vi "Undistort (Greyscale).vi"(6 "Camera Parameters":T1, 8 "error in (no error)":errorcluster, 10 "Greyscale Image Destination":T4, 11 "Greyscale Image Source":T4) -> (0 "error out":errorcluster, 3 "Greyscale Image Destination (duplicate)":T4)   [LabVIEW 2020, in "g_ar_toolkit.image.lvlib"]
uses:
  g_ar_toolkit.image.lvlib
  Greyscale Image.ctl
  g_ar_toolkit.common/Camera Parameters.ctl
  g_ar_toolkit.common/Camera Matrix.ctl
  g_ar_toolkit.common/Camera Distortion Coefficients.ctl
  88690800-d834-48c3-9c45-44dd73aae051.vi
  g_ar_toolkit.common/Module Path.vi
  <vilib>/Utility/error.llb/Error Cluster From Error Code.vi
  g_ar_toolkit.common/g_ar_toolkit.common.lvlib
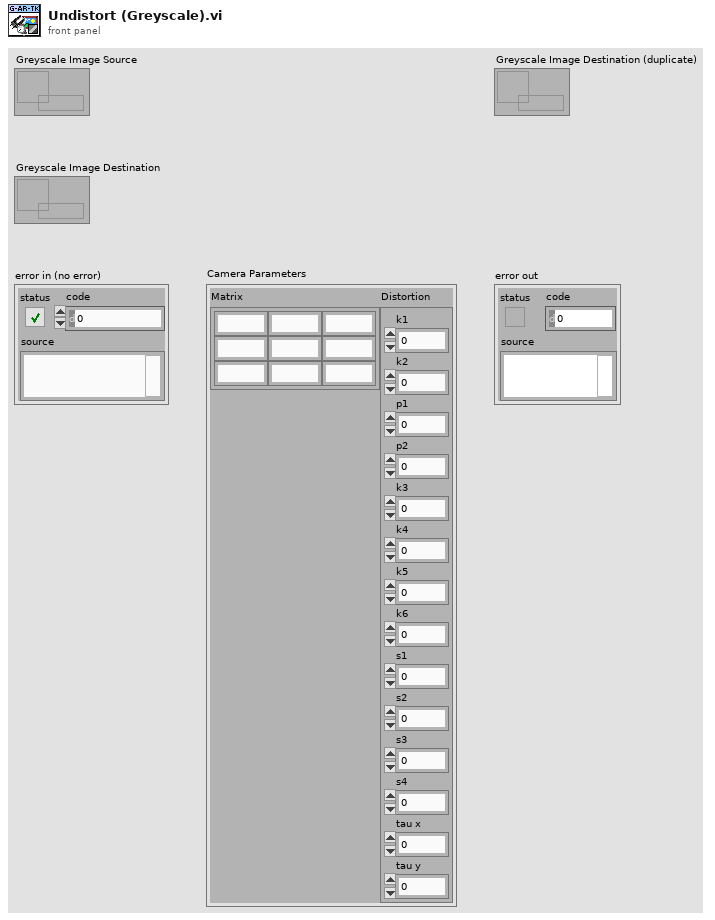
[diagram p1: front panel]
types:
  T1 = typedef "g_ar_toolkit.common.lvlib/Camera Parameters.ctl" = cluster{"Matrix":T2, "Distortion":T3}
  T2 = typedef "g_ar_toolkit.common.lvlib/Camera Matrix.ctl" = cluster{"m 0,0":dbl, "m 0,1":dbl, "m 0,2":dbl, "m 1,0":dbl, "m 1,1":dbl, "m 1,2":dbl, "m 2,0":dbl, "m 2,1":dbl, "m 2,2":dbl}
  T3 = typedef "g_ar_toolkit.common.lvlib/Camera Distortion Coefficients.ctl" = cluster{"k1":dbl, "k2":dbl, "p1":dbl, "p2":dbl, "k3":dbl, "k4":dbl, "k5":dbl, "k6":dbl, "s1":dbl, "s2":dbl, "s3":dbl, "s4":dbl, "tau x":dbl, "tau y":dbl}
  T4 = typedef "g_ar_toolkit.image.lvlib/Greyscale Image.ctl" = refnum<data-value>
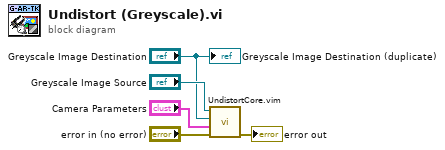
[diagram p0: block diagram]
diagram:
  n1 = call "UndistortCore.vim"("error in (no error)"="error in (no error)", "Camera Parameters"="Camera Parameters", "Dst"="Greyscale Image Destination", "Src"="Greyscale Image Source") -> ("error out"=→"error out":errorcluster)  [unwired: 7 in]
  "Greyscale Image Destination (duplicate)" <- "Greyscale Image Destination"
